vi "Plenum Fan (SubVI).vi"(11 "% Power":dbl min=0.0 max=100.0 step=1.0) -> (2 "Numeric":dbl, 3 "Required Voltage":dbl)   [LabVIEW 2019]
uses:
  <vilib>/gmath/NI_Gmath.lvlib
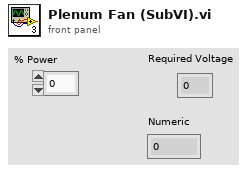
[diagram p1: front panel]
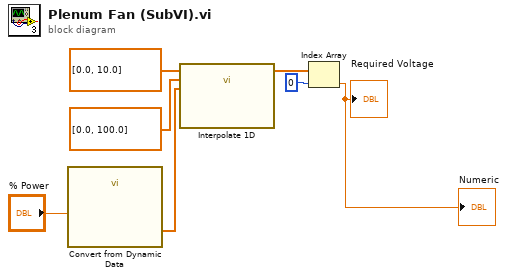
[diagram p0: block diagram]
diagram:
  n1 = call "Convert from Dynamic Data"("Dynamic Data Type"="% Power") -> ("Array"=w2:dbl[])  [unwired: 3 in]
  n2 = call <vilib>:"Interpolate 1D.vi"("xi"=w2, "X"=dbl[] [0.0, 100.0], "Y"=dbl[] [0.0, 10.0]) -> ("yi"=w1:dbl[])  [unwired: 6 in, 2 out]
  n3 = Index Array(array=w1, index=0) -> (element=→"Required Voltage" →"Numeric":dbl)
